vi "Count Of Stack.vi"(8 "error in (no error)":errorcluster caption="错误输入（无错误）", 11 "Stack 输入":refnum<class "Stack.lvclass"> caption="DNL_LabVIEW Object in") -> (0 "error out":errorcluster caption="错误输出", 2 "Count":i32, 3 "Stack 输出":refnum<class "Stack.lvclass"> caption="DNL_LabVIEW Object out")   [LabVIEW 2011, in "Stack.lvclass"]
uses:
  Stack.lvclass
  Stack.lvclass/Stack.ctl
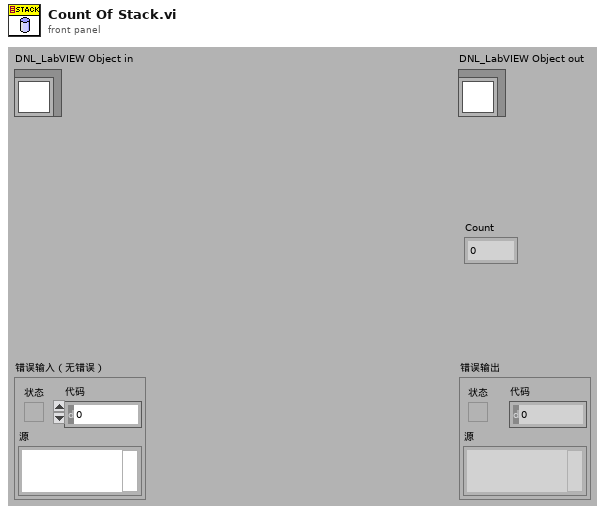
[diagram p1: front panel]
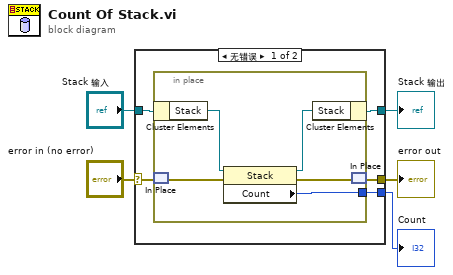
[diagram p0: block diagram]
diagram:
  n1 = case shown="无错误" "error in (no error)" {
    selector: "error in (no error)" -> [w9 w17]
    tunnel: [w8 w17] -> w4
    tunnel: [w6 w16] -> w2
    tunnel: "Stack 输入" -> [w10 w16]
    tunnel: [w7 _] -> w1
    frame No Error {
      n2 = in-place {
        in-place-border: [w11] -> w7
        n3 = in-place-cluster #1(w10) -> ("Stack"=w15:refnum<k24>)
        n4 = in-place-match #2(w9) -> (w13:errorcluster)
        n5 = property class="Stack"(reference=w15, error in=w13) -> (reference out=w14:refnum<k24>, error out=w12:errorcluster, "Count"=w11:i32)
        n6 = in-place-cluster #1("Stack"=w14) -> (w6:refnum<class "Stack.lvclass">)
        n7 = in-place-match #2(w12) -> (w8:errorcluster)
      }
    }
    frame Error {
    }
  }
  "error out" <- w4
  "Stack 输出" <- w2
  "Count" <- w1
